vi "svx_Polar_Sizes_and_Margins.vi"(5 "Selectors:Visible":bool, 7 "MagnitudeScale:Visible":bool, 9 "z scale width":u32, 11 "Container bounds":T1) -> (0 "tree top":u32, 1 "tree left":u32, 2 "tree height":u32, 3 "tree width":u32, 4 "plot area size":u32, 6 "z-scale plot height":u32)   [LabVIEW 2017, in "SVX Polar Plot.xctl"]
uses:
  <vilib>/addons/_XControls/Polar Plot/SVX Polar Plot.xctl
  <vilib>/Utility/miscctls.llb/LVBoundsTypeDef.ctl
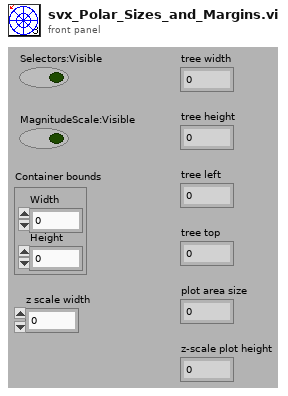
[diagram p1: front panel]
types:
  T1 = typedef "LVBoundsTypeDef.ctl" = cluster{"Width":u32, "Height":u32}
  T2 = cluster{"MARGIN_Top_Left_Bottom_Right":u32, "minimum width for visible tree control":u32, "minimum plot size":u32, "horizontal gap between z-scale and tree":i32, "horizontal gap between plot area and z-scale":i32, "Height difference from plot area to tree":u32, "vertical offset from plot area to tree":u32}
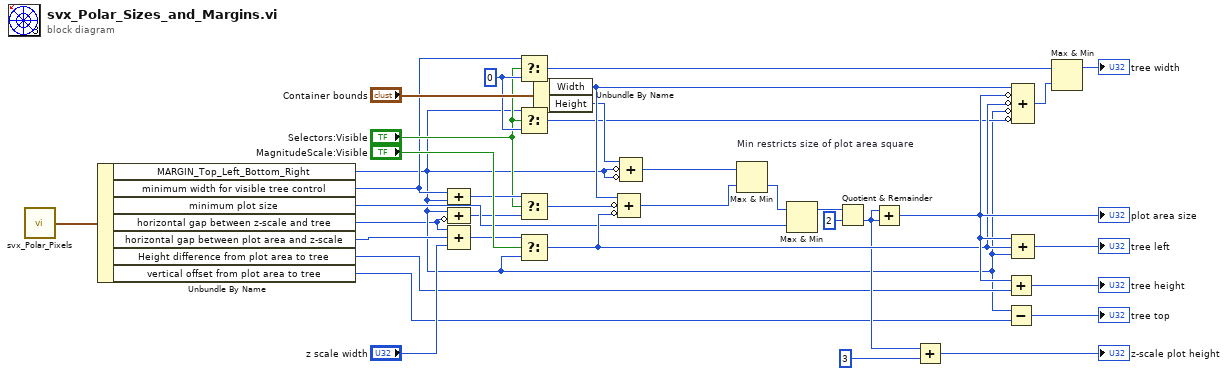
[diagram p0: block diagram]
diagram:
  w9 = u32 0 ("f")
  n1 = call <vilib>:"svx_Polar_Pixels.vi"() -> ("output cluster"=w19:T2)
  n2 = Unbundle By Name(w19) -> ("MARGIN_Top_Left_Bottom_Right"=w3:u32, "minimum width for visible tree control"=w7:u32, "minimum plot size"=w18:u32, "horizontal gap between z-scale and tree"=w1:i32, "horizontal gap between plot area and z-scale"=w14:i32, "Height difference from plot area to tree"=w13:u32, "vertical offset from plot area to tree"=w12:u32)
  n3 = Compound Arithmetic op=ADD(w7, w3) -> (w28:u32)
  n4 = Compound Arithmetic op=ADD(w3, invert w1) -> (w2:u32)
  n5 = Compound Arithmetic op=ADD(w1, w14, "z scale width") -> (w27:u32)
  n6 = Select(t=w7, s="Selectors:Visible", f=w9) -> (s? t:f=w6:u32)
  n7 = Select(t=w3, s="Selectors:Visible", f=w9) -> (s? t:f=w10:u32)
  n8 = Select(t=w28, s="Selectors:Visible", f=w2) -> (s? t:f=w11:u32)
  n9 = Select(t=w27, s="MagnitudeScale:Visible", f=w3) -> (s? t:f=w32:u32)
  n10 = Unbundle By Name("Container bounds") -> ("Width"=w26:u32, "Height"=w24:u32)
  n11 = Compound Arithmetic op=ADD(w26, invert w11, invert w32) -> (w23:u32)
  n12 = Compound Arithmetic op=ADD(w24, invert w3, invert w3) -> (w22:u32)
  n13 = Max & Min "Min restricts size of plot area square"(x=w22, y=w23) -> (min(x,y)=w17:u32)  [unwired: 1 out]
  n14 = Max & Min(x=w17, y=w18) -> (max(x,y)=w16:u32)  [unwired: 1 out]
  n15 = Quotient & Remainder(x=w16, y=u32 2) -> (floor(x/y)=w15:u32)  [unwired: 1 out]
  n16 = Add(x=w15, y=w15) -> (x+y=w33:u32)
  "plot area size" <- w33
  n17 = Add(x=w15, y=u32 3 ("x")) -> (x+y=→"z-scale plot height":u32)
  n18 = Add(x=w33, y=w13) -> (x+y=→"tree height":u32)
  n19 = Subtract(x=w3, y=w12) -> (x-y=→"tree top":u32)
  n20 = Compound Arithmetic op=ADD(w26, invert w33, invert w32, invert w3, invert w10) -> (w5:u32)
  n21 = Compound Arithmetic op=ADD(w33, w32, w3) -> (→"tree left":u32)
  n22 = Max & Min(x=w6, y=w5) -> (max(x,y)=→"tree width":u32)  [unwired: 1 out]
